vi "ADC X-jalg.vi"() -> ()   [LabVIEW 2012]
uses:
  <vilib>/Waveform/WDTFileIO.llb/ Write Waveform to File.vi
  <vilib>/Analysis/NI_AALBase.lvlib
panel:
  in  "rate":dbl=10000.0
  in  "number of samples":i32=400
  in  "stop":bool
  out "Time Elapsed":dbl=548.319
  out "Samples per Second":dbl=20.001130728645187
  out "Waveform Graph":waveform(dbl)(graph)={"t0"=timestamp(0 s since 1904-01-01), "dt"=0.05, "Y"=array[10967 elements]}
  in  "Write to file?":bool
  in  "file path (dialog if empty)":path
  in  "Append to file?":bool
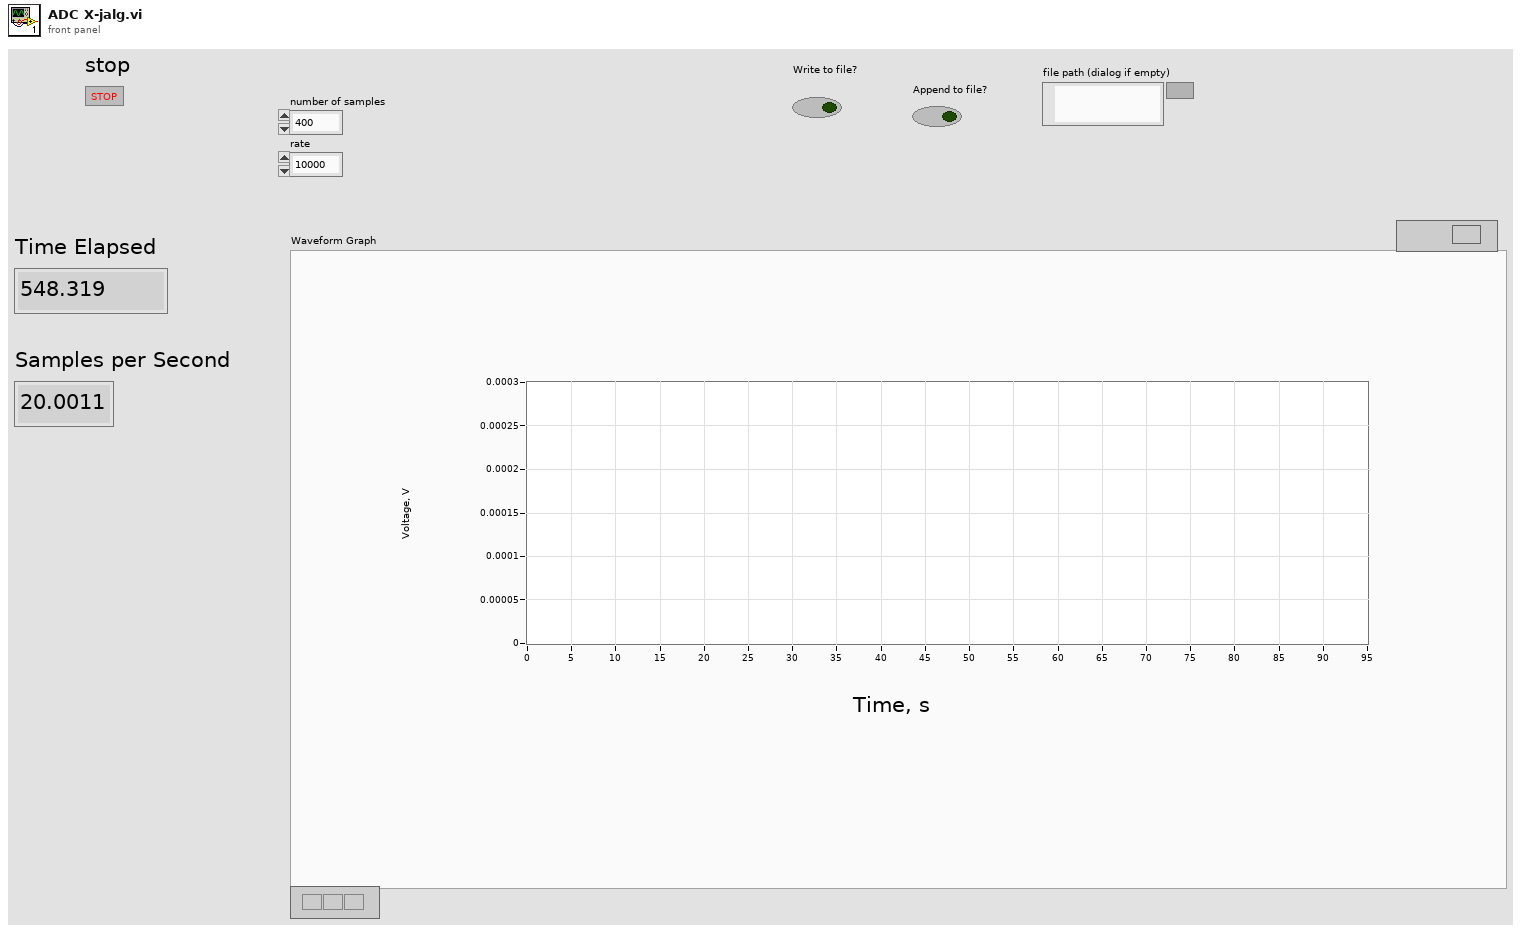
[diagram p1: front panel]
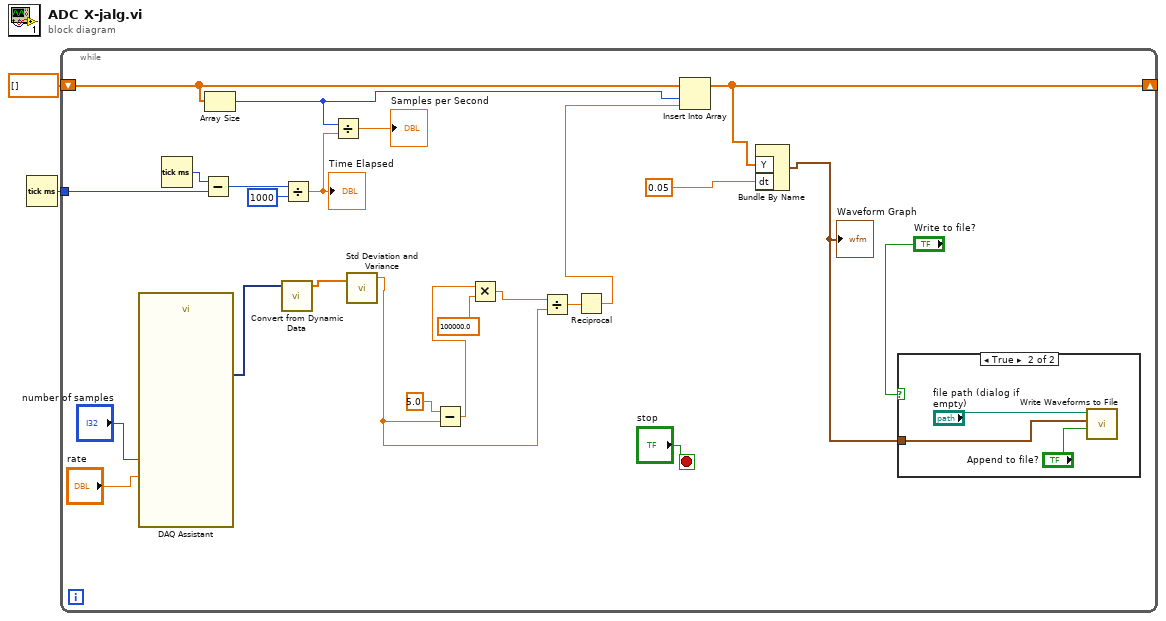
[diagram p0: block diagram]
diagram:
  n1 = Tick Count (ms)() -> (millisecond timer value=w1:u32)
  n2 = while {
    shift-right: [w12] -> _
    shift-left: dbl[] [] -> [w21]
    tunnel: w1 -> [w24]
    stop <- "stop" stop-if-true
    n3 = call "DAQ Assistant"("rate"="rate", "number of samples"="number of samples") -> ("data"=w17:dynamicdata)  [unwired: 15 in, 2 out]
    n4 = Tick Count (ms)() -> (millisecond timer value=w25:u32)
    n5 = Subtract(x=w25, y=w24) -> (x-y=w23:u32)
    n6 = Array Size(array=w21) -> (size(s)=w18:i32)
    n7 = call "Convert from Dynamic Data"("Dynamic Data Type"=w17) -> ("Array"=w9:dbl[])  [unwired: 3 in]
    n8 = Divide(x=w23, y=u32 1000) -> (x/y=w20:dbl)
    "Time Elapsed" <- w20
    n9 = Divide(x=w18, y=w20) -> (x/y=→"Samples per Second":dbl)
    n10 = call <vilib>:"Std Deviation and Variance.vi"("X"=w9) -> ("mean"=w5:dbl)  [unwired: 1 in, 2 out]
    n11 = Subtract(x=5.0, y=w5) -> (x-y=w6:dbl)
    n12 = Multiply(x=w6, y=100000.0) -> (x*y=w10:dbl)
    n13 = Divide(x=w10, y=w5) -> (x/y=w4:dbl)
    n14 = Reciprocal(x=w4) -> (1/x=w3:dbl)
    n15 = Insert Into Array(array=w21, index=w18, new element=w3) -> (w12:dbl[])
    n16 = Bundle By Name("Y"=w12, "dt"=0.05 ("1/x")) -> (w11:waveform(dbl))  [unwired: 1 in]
    "Waveform Graph" <- w11
    n17 = case shown="True" "Write to file?" {
      tunnel: w11 -> [_ w27]
      frame False {
      }
      frame True {
        n18 = call-poly <vilib>:"Write Waveforms to File.vi"("append to file? (new file:F)"="Append to file?", "waveform"=w27, "file path (dialog if empty)"="file path (dialog if empty)") -> ()  [unwired: 7 in, 2 out]
      }
    }
  }
